vi "Finish.vi"(8 "error in (no error)":errorcluster, 11 "Catapult in":refnum<class "Catapult.lvclass">) -> (0 "error out":errorcluster, 3 "Catapult out":refnum<class "Catapult.lvclass">)   [LabVIEW 2013, in "Catapult.lvclass"]
uses:
  Catapult.lvclass
  System/System.lvclass
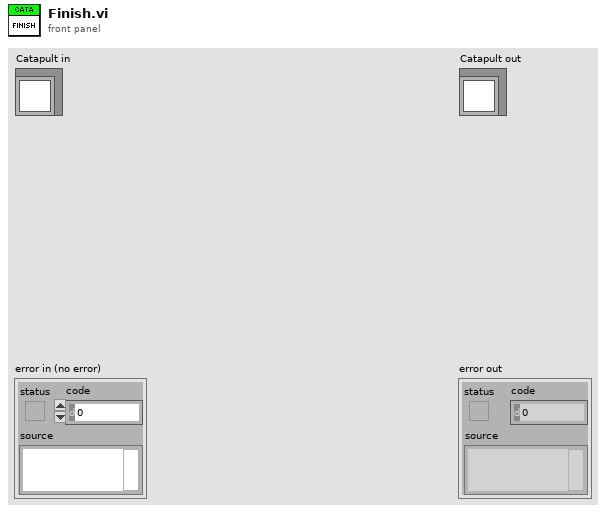
[diagram p1: front panel]
types:
  T1 = typedef "WPI_DigitalInputDevRef.ctl" = cluster{"DevStatus":errorcluster, "DIO Channel":T2, "Digital Module":T3}
  T2 = typedef "FPGA_DIOChannel.ctl" = enum8{"DIO 1", "DIO 2", "DIO 3", "DIO 4", "DIO 5", "DIO 6", "DIO 7", "DIO 8", "DIO 9", "DIO 10", "DIO 11", "DIO 12", "DIO 13", "DIO 14", "Invalid"}
  T3 = typedef "FPGA_TypedefDigitalModule.ctl" = enum16{"Digital Module 1", "Digital Module 2"}
  T4 = typedef "WPI_MotorControlDeviceRef.ctl" = cluster{"DeviceStatus":errorcluster, "Type":enum16{"PWM", "CAN"}, "PWM":cluster{"Digital Module":T3, "PWM Channel":T5, "DeadBand":T6}, "CAN":cluster{"Device Number":u8, "Control Mode":T7, "Semaphore":T8, "Max Vout":dbl}, "Invert":bool, "TransformRef":T9, "InvTransformRef":T9}
  T5 = typedef "FPGA_DIOPWMChannel.ctl" = enum8{"PWM 1", "PWM 2", "PWM 3", "PWM 4", "PWM 5", "PWM 6", "PWM 7", "PWM 8", "PWM 9", "PWM 10", "Invalid"}
  T6 = typedef "WPI_PWMDeadband.ctl" = cluster{"Name":string, "maxPositivePwm":i32, "minPositivePwm":i32, "centerPwm":i32, "maxNegativePwm":i32, "minNegativePwm":i32, "angularRange":u16}
  T7 = typedef "WPI_CANJaguar_ControlMode.ctl" = enum8{"Percent VBus", "Current", "Speed", "Position", "Voltage"}
  T8 = typedef "Semaphore RefNum" = refnum<k1>
  T9 = typedef "WPI_PWMTransform_ConPane.ctl" = refnum<vi>
  T10 = typedef "WPI_SolenoidDevRef.ctl" = cluster{"DevStatus":errorcluster, "Solenoid Module":T11, "Forward Solenoid Channel":T12, "Reverse Solenoid Channel":T12}
  T11 = typedef "FPGA_TypedefSolenoidModule.ctl" = enum16{"Solenoid Module 1", "Solenoid Module 2"}
  T12 = typedef "WPI_SolenoidChannel.ctl" = enum8{"Solenoid 1", "Solenoid 2", "Solenoid 3", "Solenoid 4", "Solenoid 5", "Solenoid 6", "Solenoid 7", "Solenoid 8", "Invalid"}
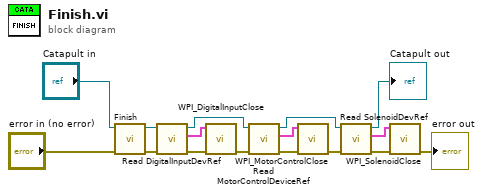
[diagram p0: block diagram]
diagram:
  n1 = call-parent "Finish.vi"("error in (no error)"="error in (no error)", "System in"="Catapult in") -> ("error out"=w2:errorcluster, "System out"=w14:refnum<class "Catapult.lvclass">)  [unwired: 8 in]
  n2 = call-dynamic "Read DigitalInputDevRef.vi"("error in (no error)"=w2, "Catapult in"=w14) -> ("error out"=w7:errorcluster, "DigitalInputDevRef"=w13:T1, "Catapult out"=w12:refnum<class "Catapult.lvclass">)  [unwired: 7 in]
  n3 = call <vilib>:"WPI_DigitalInputClose.vi"("error in (no error)"=w7, "DigitalInputDevRef"=w13) -> ("error out"=w6:errorcluster)  [unwired: 9 in]
  n4 = call-dynamic "Read MotorControlDeviceRef.vi"("error in (no error)"=w6, "Catapult in"=w12) -> ("error out"=w5:errorcluster, "MotorControlDeviceRef"=w11:T4, "Catapult out"=w10:refnum<class "Catapult.lvclass">)  [unwired: 7 in]
  n5 = call <vilib>:"WPI_MotorControlClose.vi"("error in (no error)"=w5, "MotorControlDevRef"=w11) -> ("error out"=w4:errorcluster)  [unwired: 9 in]
  n6 = call-dynamic "Read SolenoidDevRef.vi"("error in (no error)"=w4, "Catapult in"=w10) -> ("error out"=w3:errorcluster, "SolenoidDevRef"=w8:T10, "Catapult out"=→"Catapult out":refnum<class "Catapult.lvclass">)  [unwired: 7 in]
  n7 = call <vilib>:"WPI_SolenoidClose.vi"("error in (no error)"=w3, "SolenoidDevRef"=w8) -> ("error out"=→"error out":errorcluster)  [unwired: 9 in]
